vi "back to base.vi"   [LabVIEW 2018]
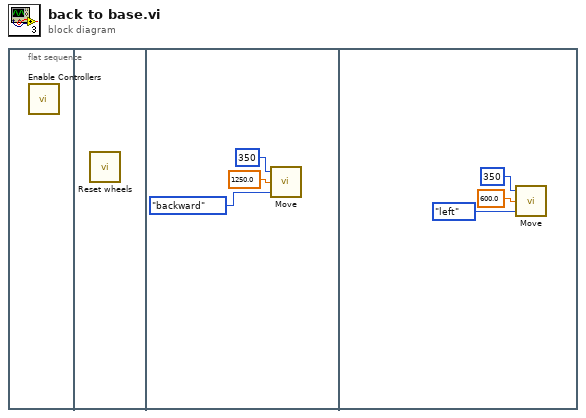
[diagram p0: block diagram]
diagram:
  n1 = flat-sequence {
    frame #0 {
      n2 = call "Enable Controllers.vi"() -> ()  [unwired: 12 in]
    }
    frame #1 {
      n3 = call "Reset wheels.vi"() -> ()  [unwired: 12 in]
    }
    frame #2 {
      n4 = call "Move.vi"("Enum"=enum16{"forward", "backward", "left", "right"}."backward", "distance"=1250.0, "speed"=350) -> ()  [unwired: 1 in]
    }
    frame #3 {
      n5 = call "Move.vi"("Enum"=enum16{"forward", "backward", "left", "right"}."left", "distance"=600.0, "speed"=350) -> ()  [unwired: 1 in]
    }
  }
